vi "Ramp Slow.vi"(8 "error in (no error)":errorcluster, 9 "fieldIN":dbl[unit] caption="Field", 10 "Rate":dbl[unit], 11 "Power Supply in":refnum<class "Power Supply.lvclass">) -> (0 "error out":errorcluster, 1 "Rate Out":dbl[unit], 3 "Power Supply out":refnum<class "Power Supply.lvclass">)   [LabVIEW 2009, in "Power Supply.lvclass"]
uses:
  Power Supply.lvclass
  Power Supply.lvclass/Power Supply.ctl
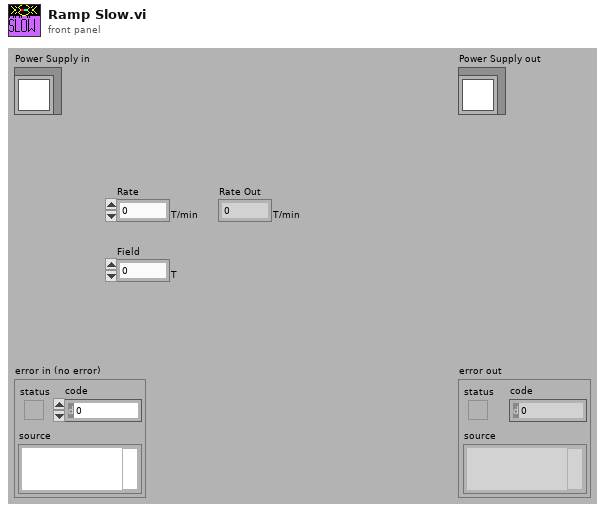
[diagram p1: front panel]
types:
  T1 = typedef "PSIO.ctl" = cluster{"Address":T2, "Version":enum16{"PS", "IPS"}}
  T2 = typedef "OxfordAddress.ctl" = cluster{"Com Port":i32, "ISOBUS Address":i32, "GPIB Address":i16, "Communication":enum16{"RS232", "ISOBUS", "GPIB", "Gateway"}}
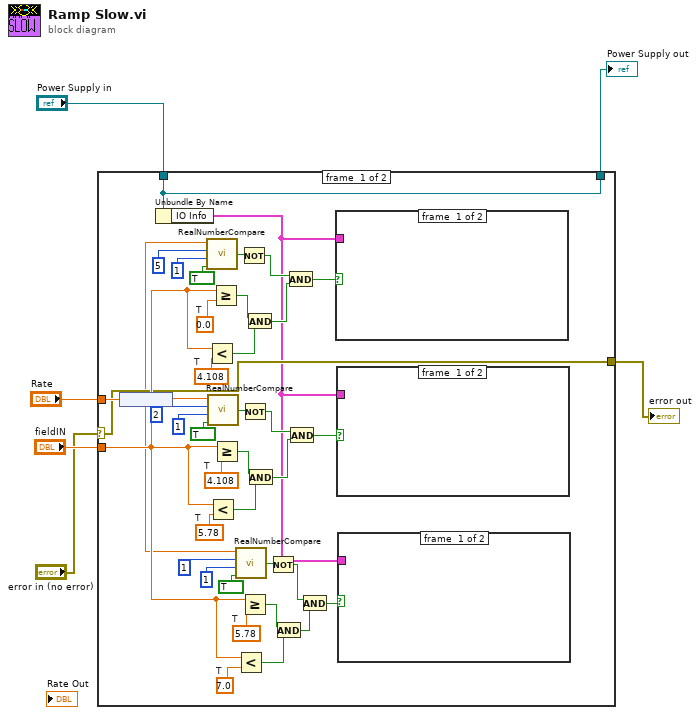
[diagram p0: block diagram]
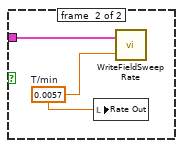
[diagram p2: hidden frame]
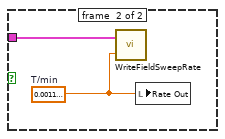
[diagram p3: hidden frame]
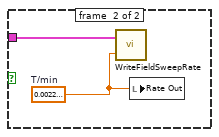
[diagram p4: hidden frame]
diagram:
  n1 = case shown="No Error" "error in (no error)" {
    selector: "error in (no error)" -> [w10 w52]
    tunnel: "fieldIN" -> [w45 _]
    tunnel: "Rate" -> [w44 _]
    tunnel: [w10 w52] -> w3
    tunnel: "Power Supply in" -> [w8 w53]
    tunnel: [w8 w53] -> w1
    frame #0 {
      w16 = dbl[unit] 4.108  # T
      w21 = dbl[unit] 0.0  # T
      w27 = dbl[unit] 7.0  # T
      w32 = dbl[unit] 5.78  # T
      w37 = dbl[unit] 5.78  # T
      w43 = dbl[unit] 4.108  # T
      n2 = node(w44) -> (w7:dbl)
      n3 = Unbundle By Name(w8) -> ("IO Info"=w9:T1)
      n4 = call "RealNumberCompare.vi"("Percent? (Default F)"=TRUE, "Difference?"=1, "Number 2"=5, "Number 1"=w7) -> ("Equal to?"=w20:bool)
      n5 = Less?(x=w45, y=w16) -> (x < y?=w14:bool)
      n6 = call "RealNumberCompare.vi"("Percent? (Default F)"=TRUE, "Difference?"=1, "Number 2"=2, "Number 1"=w7) -> ("Equal to?"=w41:bool)
      n7 = Less?(x=w45, y=w37) -> (x < y?=w35:bool)
      n8 = Greater Or Equal?(x=w45, y=w21) -> (x >= y?=w15:bool)
      n9 = Greater Or Equal?(x=w45, y=w43) -> (x >= y?=w36:bool)
      n10 = call "RealNumberCompare.vi"("Percent? (Default F)"=TRUE, "Difference?"=1, "Number 2"=1, "Number 1"=w7) -> ("Equal to?"=w30:bool)
      n11 = Less?(x=w45, y=w27) -> (x < y?=w25:bool)
      n12 = Not(x=w20) -> (.not. x?=w19:bool)
      n13 = Not(x=w41) -> (.not. x?=w40:bool)
      n14 = Greater Or Equal?(x=w45, y=w32) -> (x >= y?=w26:bool)
      n15 = And(x=w15, y=w14) -> (x .and. y?=w13:bool)
      n16 = And(x=w36, y=w35) -> (x .and. y?=w34:bool)
      n17 = Not(x=w30) -> (.not. x?=w24:bool)
      n18 = And(x=w26, y=w25) -> (x .and. y?=w23:bool)
      n19 = And(x=w19, y=w13) -> (x .and. y?=w12:bool)
      n20 = And(x=w40, y=w34) -> (x .and. y?=w33:bool)
      n21 = And(x=w24, y=w23) -> (x .and. y?=w22:bool)
      n22 = case shown="True" w12 {
        tunnel: w9 -> [_ w47]
        frame #0 {
        }
        frame #1 {
          w46 = dbl[unit] 0.0057  # T/min
          n23 = local write "Rate Out"(w46) -> ()
          n24 = call "WriteFieldSweepRate.vi"("Sweep rate"=w46, "IO Info"=w47) -> ()  [unwired: 1 out]
        }
      }
      n25 = case shown="True" w33 {
        tunnel: w9 -> [_ w51]
        frame #0 {
        }
        frame #1 {
          w50 = dbl[unit] 0.0022833333333333334  # T/min
          n26 = call "WriteFieldSweepRate.vi"("Sweep rate"=w50, "IO Info"=w51) -> ()  [unwired: 1 out]
          n27 = local write "Rate Out"(w50) -> ()
        }
      }
      n28 = case shown="True" w22 {
        tunnel: w9 -> [_ w49]
        frame #0 {
        }
        frame #1 {
          w48 = dbl[unit] 0.0011333333333333334  # T/min
          n29 = call "WriteFieldSweepRate.vi"("Sweep rate"=w48, "IO Info"=w49) -> ()  [unwired: 1 out]
          n30 = local write "Rate Out"(w48) -> ()
        }
      }
    }
    frame #1 {
    }
  }
  "error out" <- w3
  "Power Supply out" <- w1
